vi "WPI_DashboardVIdeo Path for Read.vi"(11 "Display Name":string) -> (3 "Video Path":path)   [LabVIEW 2017]
uses:
  <vilib>/Rock Robotics/WPI/Dashboard/WPI_DashboardLogging Global.vi
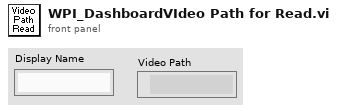
[diagram p1: front panel]
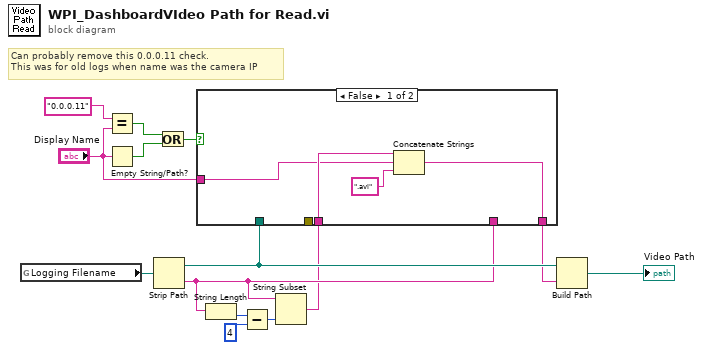
[diagram p0: block diagram]
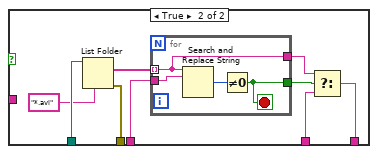
[diagram p2: hidden frame]
diagram:
  # "Can probably remove this 0.0.0.11 check.\nThis was for old logs when name was the camera IP"
  n1 = global read "WPI_DashboardLogging Global.vi" "Logging Filename"() -> (w14:path)
  n2 = Equal?(x="0.0.0.11", y="Display Name") -> (x = y?=w3:bool)
  n3 = Empty String/Path?(string/path="Display Name") -> (empty?=w2:bool)
  n4 = Strip Path(path=w14) -> (stripped path=w12:path, name=w8:string)
  n5 = Or(x=w3, y=w2) -> (x .or. y?=w1:bool)
  n6 = String Length(string=w8) -> (length=w9:i32)
  n7 = Subtract(x=w9, y=4) -> (x-y=w7:i32)
  n8 = String Subset(string=w8, length (rest)=w7) -> (substring=w6:string)  [unwired: 1 in]
  n9 = case shown="False" w1 {
    tunnel: w12 -> [_ w27]
    tunnel: [w15 w22] -> w11
    tunnel: w8 -> [_ w21]
    tunnel: w6 -> [w18 w20]
    tunnel: "Display Name" -> [w17 _]
    tunnel: [_ w19] -> _
    frame False {
      n10 = Concatenate Strings(w18, w17, ".avi") -> (w15:string)
    }
    frame True {
      n11 = List Folder(path=w27, pattern="*.avi") -> (filenames=w26:string[], error out=w19:errorcluster)  [unwired: 2 in, 2 out]
      n12 = for {
        tunnel: w26 -> [w29] mode=indexing
        tunnel: w20 -> [w31]
        tunnel: [w29] -> w23
        tunnel: [w28] -> w24
        stop <- w28 stop-if-true
        n13 = Search and Replace String(input string=w29, search string=w31) -> (number of replacements=w30:i32)  [unwired: 6 in, 3 out]
        n14 = Not Equal To 0?(x=w30) -> (x != 0?=w28:bool)
      }
      n15 = Select(t=w23, s=w24, f=w21) -> (s? t:f=w22:string)
    }
  }
  n16 = Build Path(base path=w12, name or relative path=w11) -> (appended path=→"Video Path":path)
